vi "Read XML.vi"(8 "error in":errorcluster, 11 "path":path) -> (0 "error out":errorcluster, 1 "StepObj Out":refnum<class "STEP.lvclass">[](array[class]), 2 "Steps":string[](array[string]), 3 "Values":string[](array[string]), 5 "tags":string[](array[string]))   [LabVIEW 2015]
uses:
  Reusable/Sequence/STEPS/STEP.lvclass
  <vilib>/xml/Load XML File.vi
  <vilib>/xml/Close Reference(Node).vi
  <vilib>/xml/Close Reference(NdList).vi
  <vilib>/xml/NI_XML.lvlib
  <resource>/objmgr/DOMUserDefRef.rc
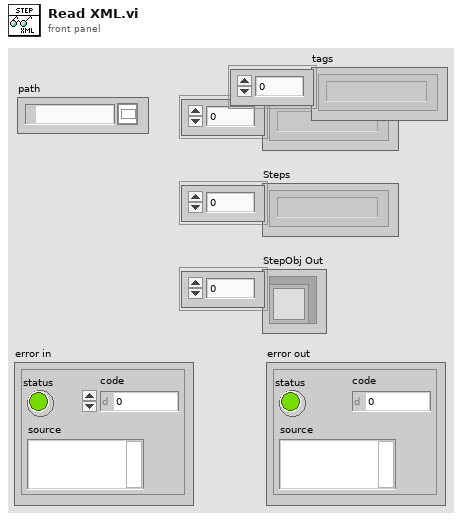
[diagram p1: front panel]
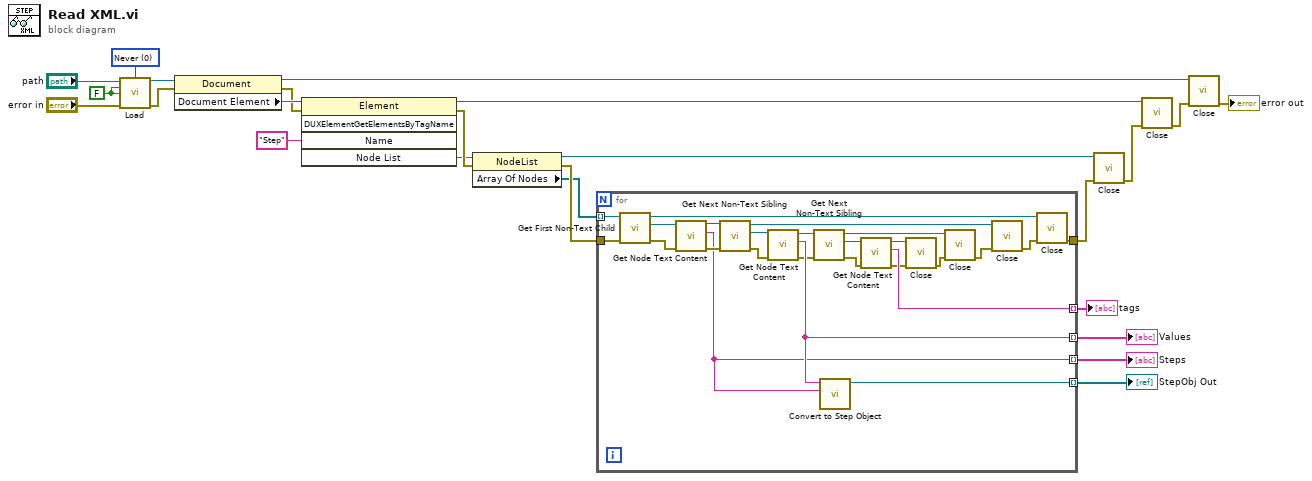
[diagram p0: block diagram]
diagram:
  w5 = 0 items=["Never", "Always", "Auto"] ("Validate On Load")
  w3 = FALSE ("Do Namespaces")
  n1 = call-poly <vilib>:"Load.vi"("path to XML document"="path", "validate on load (Auto)"=w5, "process namespaces (False)"=w3, "process schema (False)"=w3, "error in (no error)"="error in") -> ("DOM document out"=w9:refnum<k20>, "error out"=w10:errorcluster)  [unwired: 2 in, 7 out]
  n2 = property class="Document"(reference=w9, error in=w10) -> (reference out=w18:refnum<k20>, error out=w6:errorcluster, "Document Element"=w7:refnum<k20>)
  n3 = invoke class="Element" method="DUXElementGetElementsByTagName"(reference=w7, error in=w6, "Name"="Step" ("Node Name")) -> (reference out=w15:refnum<k20>, error out=w22:errorcluster, "Node List"=w11:refnum<k20>)  [unwired: 2 in, 2 out]
  n4 = property class="NodeList"(reference=w11, error in=w22) -> (reference out=w13:refnum<k20>, error out=w23:errorcluster, "Array Of Nodes"=w12:refnum<k20>[])
  n5 = for {
    tunnel: w12 -> [w43] mode=indexing
    tunnel: [w38] -> w14
    tunnel: [w36] -> w19 mode=indexing
    tunnel: [w35] -> w20 mode=indexing
    tunnel: w23 -> [w37]
    tunnel: [w34] -> w24 mode=indexing
    tunnel: [w29] -> w1 mode=indexing
    n6 = call <vilib>:"Get First Non-Text Child.vi"("error in (no error)"=w37, "node in"=w43) -> ("error out"=w45:errorcluster, "child node"=w44:refnum<k20>, "node out"=w39:refnum<k20>)  [unwired: 7 out]
    n7 = call <vilib>:"Get Node Text Content.vi"("error in (no error)"=w45, "node in"=w44) -> ("error out"=w49:errorcluster, "node text"=w35:string, "node out"=w48:refnum<k20>)  [unwired: 7 out]
    n8 = call <vilib>:"Get Next Non-Text Sibling.vi"("error in (no error)"=w49, "node in"=w48) -> ("error out"=w46:errorcluster, "sibling node"=w47:refnum<k20>, "node out"=w41:refnum<k20>)  [unwired: 7 out]
    n9 = call <vilib>:"Get Node Text Content.vi"("error in (no error)"=w46, "node in"=w47) -> ("error out"=w33:errorcluster, "node text"=w36:string, "node out"=w32:refnum<k20>)  [unwired: 7 out]
    n10 = call <vilib>:"Get Next Non-Text Sibling.vi"("error in (no error)"=w33, "node in"=w32) -> ("error out"=w30:errorcluster, "sibling node"=w31:refnum<k20>, "node out"=w25:refnum<k20>)  [unwired: 7 out]
    n11 = call "Convert to Step Object.vi"("Step"=w35, "Value"=w36) -> ("STEP out"=w34:refnum<class "STEP.lvclass">)  [unwired: 8 in, 1 out]
    n12 = call <vilib>:"Get Node Text Content.vi"("error in (no error)"=w30, "node in"=w31) -> ("error out"=w27:errorcluster, "node text"=w29:string, "node out"=w28:refnum<k20>)  [unwired: 7 out]
    n13 = call-poly <vilib>:"Close.vi"("error in (no error)"=w27, "node"=w28) -> ("error out"=w26:errorcluster)  [unwired: 7 out]
    n14 = call-poly <vilib>:"Close.vi"("error in (no error)"=w26, "node"=w25) -> ("error out"=w42:errorcluster)  [unwired: 7 out]
    n15 = call-poly <vilib>:"Close.vi"("error in (no error)"=w42, "node"=w41) -> ("error out"=w40:errorcluster)  [unwired: 7 out]
    n16 = call-poly <vilib>:"Close.vi"("error in (no error)"=w40, "node"=w39) -> ("error out"=w38:errorcluster)  [unwired: 7 out]
  }
  "Values" <- w19
  "Steps" <- w20
  "StepObj Out" <- w24
  "tags" <- w1
  n17 = call-poly <vilib>:"Close.vi"("error in (no error)"=w14, "node list"=w13) -> ("error out"=w16:errorcluster)  [unwired: 7 out]
  n18 = call-poly <vilib>:"Close.vi"("error in (no error)"=w16, "node"=w15) -> ("error out"=w17:errorcluster)  [unwired: 7 out]
  n19 = call-poly <vilib>:"Close.vi"("error in (no error)"=w17, "node"=w18) -> ("error out"=→"error out":errorcluster)  [unwired: 7 out]
